vi "Get_Intensity_Value_For_Thresholding-1.vi"(0 "[IN] Index of starting \npoint for thresholding":i32, 1 "[IN] Thresholding range":cluster{"Lower value":sgl, "Upper value":sgl}={"Lower value"=128.0, "Upper value"=255.0}, 3 "error IN":errorcluster, 4 "[IN] Index for \nthresholding":u8) -> (5 "[OUT] Thresholding range":cluster{"Lower value":sgl, "Upper value":sgl}, 6 "error OUT":errorcluster)   [LabVIEW 2013]
doc: "SubVI saves used for thresholding limits (255 - commonly highest value, user defines only 1 value for threshold)"
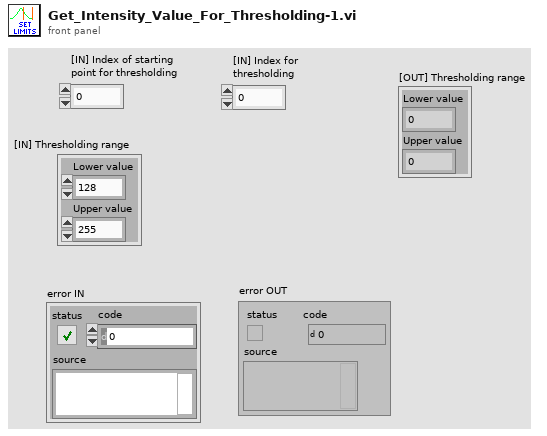
[diagram p1: front panel]
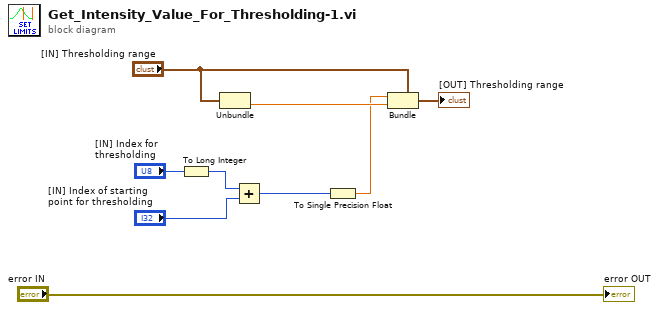
[diagram p0: block diagram]
diagram:
  n1 = To Long Integer(number="[IN] Index for \nthresholding") -> (32bit integer=w7:i32)
  n2 = Unbundle("[IN] Thresholding range") -> ("Upper value"=w5:sgl)  [unwired: 1 out]
  n3 = Add(x=w7, y="[IN] Index of starting \npoint for thresholding") -> (x+y=w1:i32)
  n4 = To Single Precision Float(number=w1) -> (single precision float=w4:sgl)
  n5 = Bundle(cluster="[IN] Thresholding range", "Lower value"=w4, "Upper value"=w5) -> (→"[OUT] Thresholding range":cluster{"Lower value":sgl, "Upper value":sgl})
  "error OUT" <- "error IN"
